vi "6517b.vi"(11 "VISA resource name":refnum<visa-resource-name>="GPIB0::12::INSTR") -> ()   [LabVIEW 2019]
uses:
  <vilib>/Utility/file.llb/Write To Spreadsheet File (DBL).vi
  lib/Keithley 6517/Keithley 6517.lvlib
panel:
  in  "Voltage Source Level (0.000000E+0)":dbl=2.0 format="%#_13g"
  in  "VISA resource name":refnum<visa-resource-name>
  in  "采集最小间隔（ms）":u32
  out "date/time string":string="20171114204549"
  in  "file path (dialog if empty)":path
  # "K"
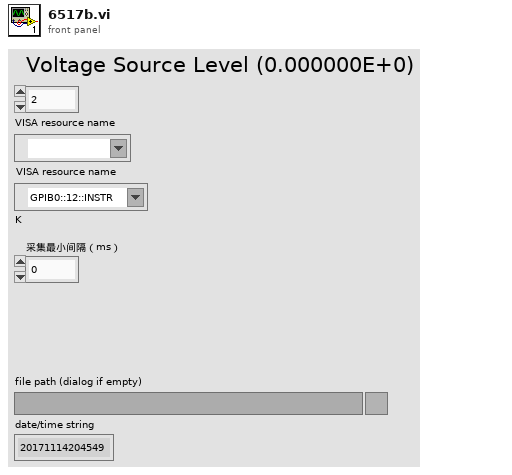
[diagram p1: front panel]
types:
  T1 = enum16{"open", "replace", "create", "open or create", "replace or create", "replace or create with confirmation"}
  T2 = cluster{"Measurement":dbl, "Units":string, "Time Stamp and Date":string, "Reading #":dbl, "Channel #":dbl}
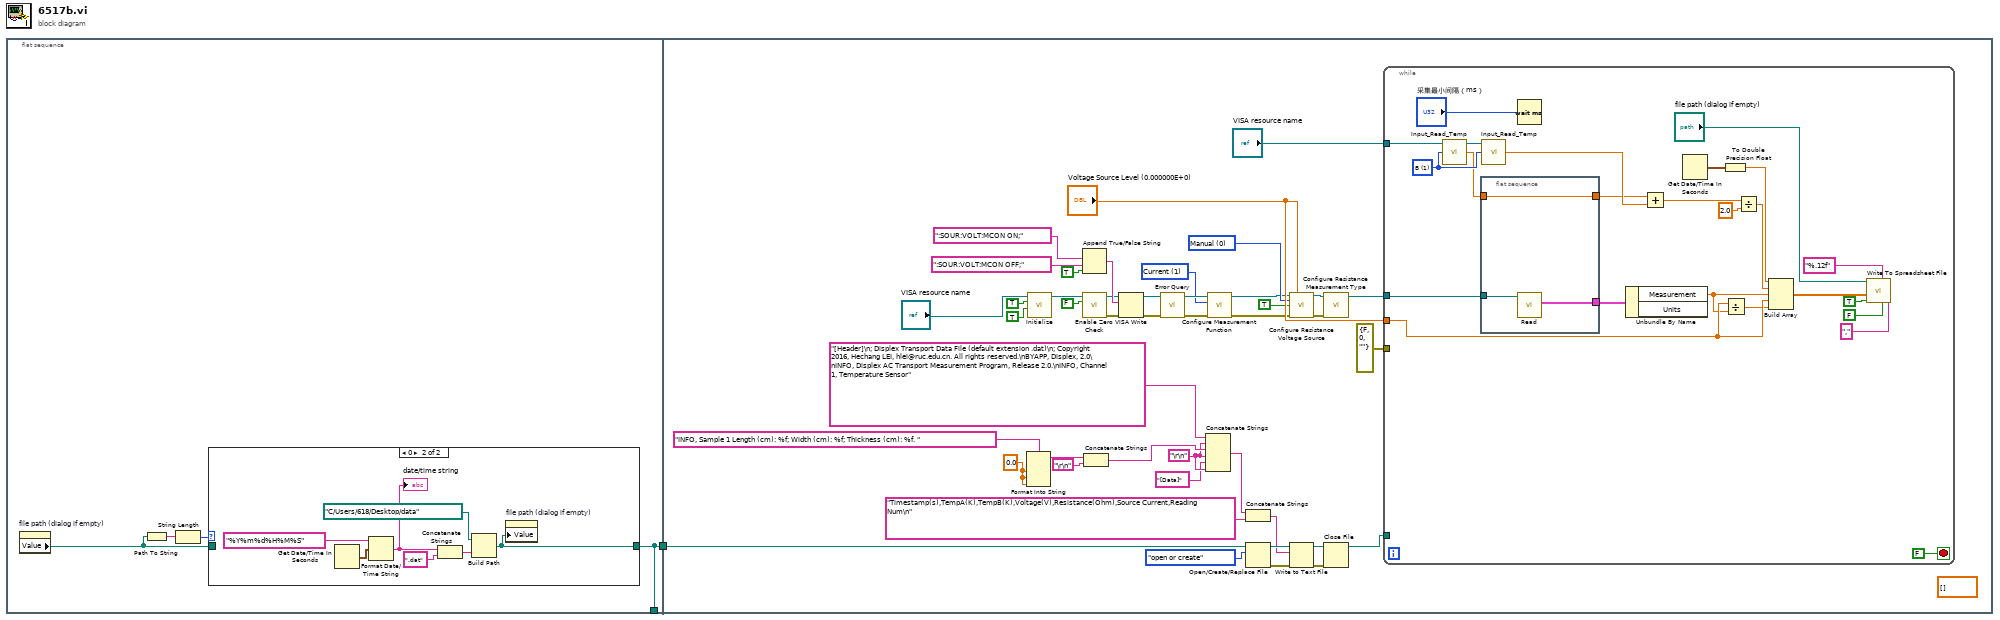
[diagram p0: block diagram]
diagram:
  n1 = flat-sequence {
    tunnel: [w2] -> _
    tunnel: [w2] -> w1
    tunnel: w1 -> [w55]
    frame #0 {
      n2 = property on="file path (dialog if empty)" class="Path"() -> ("Value"=w3:path)  [unwired: 2 in, 2 out]
      n3 = Path To String(path=w3) -> (string=w5:string)
      n4 = String Length(string=w5) -> (length=w4:i32)
      n5 = case shown="0" w4 {
        tunnel: [w6 w7] -> w2
        tunnel: w3 -> [w6 _]
        frame 1, Default {
        }
        frame 0 {
          n6 = Get Date/Time In Seconds() -> (seconds since 1Jan1904=w13:timestamp)
          n7 = Format Date/Time String(time format string (%c)="%Y%m%d%H%M%S", seconds (now)=w13) -> (date/time string=w8:string)  [unwired: 1 in]
          "date/time string" <- w8
          n8 = Concatenate Strings(w8, ".dat" ("string")) -> (w9:string)
          n9 = Build Path(base path=path "C:/Users/618/Desktop/data" ("文件夹路径"), name or relative path=w9) -> (appended path=w7:path)
          n10 = property on="file path (dialog if empty)" class="Path"("Value"=w7) -> ()  [unwired: 2 in, 2 out]
        }
      }
    }
    frame #1 {
      w18 = 1 items=["Voltage", "Current", "Resistance", "Charge"] ("Measurement Function (0: Voltage)")
      w24 = 0 items=["Manual", "Auto"] ("Voltage Source Mode (0: Manual)")
      w44 = 0.0 ("输入 1")
      w47 = "\r\n"
      (unwired) dbl[] []
      n11 = Format Into String(format string="INFO, Sample 1 Length (cm): %f; Width (cm): %f; Thickness (cm): %f. " ("string"), w44, w44, w44) -> (resulting string=w51:string)  [unwired: 2 in, 1 out]
      n12 = call "Initialize.vi"("Reset (True)"=TRUE, "ID Query (True)"=TRUE, "VISA resource name"="VISA resource name") -> ("VISA resource name out"=w16:refnum<visa-resource-name>)  [unwired: 7 in, 1 out]
      n13 = Append True/False String(1:TRUE ("Enable LO Connection (F: Disable)"), 2:":SOUR:VOLT:MCON OFF;", 3:":SOUR:VOLT:MCON ON;") -> (0:w32:string)  [unwired: 1 in]
      n14 = call "Enable Zero Check.vi"("Enable Zero Check (T: Enable)"=FALSE, "VISA resource name"=w16) -> ("error out"=w30:errorcluster, "VISA resource name out"=w31:refnum<visa-resource-name>)  [unwired: 8 in]
      n15 = Concatenate Strings(w51, "\r\n") -> (w52:string)
      n16 = VISA Write(VISA resource name=w31, write buffer=w32, error in (no error)=w30) -> (VISA resource name out=w29:refnum<visa-resource-name>, error out=w28:errorcluster)  [unwired: 1 out]
      n17 = call "Error Query.vi"("error in (no error)"=w28, "VISA resource name"=w29) -> ("error out"=w22:errorcluster, "VISA resource name out"=w21:refnum<visa-resource-name>)  [unwired: 6 in, 2 out]
      n18 = Concatenate Strings("[Header]\n; Displex Transport Data File (default extension .dat)\n; Copyright 2016, Hechang LEI, hlei@ruc.edu.cn. All rights reserved.\nBYAPP, Displex, 2.0\nINFO, Displex AC Transport Measurement Program, Release 2.0.\nINFO, Channel 1, Temperature Sensor" ("string"), w47, w52, w47, "[Data]" ("string"), w47) -> (w53:string)
      n19 = call "Configure Measurement Function.vi"("error in (no error)"=w22, "Measurement Function (0: Voltage)"=w18, "VISA resource name"=w21) -> ("error out"=w19:errorcluster, "VISA resource name out"=w20:refnum<visa-resource-name>)  [unwired: 7 in]
      n20 = Concatenate Strings(w53, "Timestamp(s),TempA(K),TempB(K),Voltage(V),Resistance(Ohm),Source Current,Reading Num\n" ("字符串")) -> (w43:string)
      n21 = Open/Create/Replace File(file path (use dialog)=w55, operation (0:open)=T1."open or create") -> (refnum out=w54:refnum<file>, error out=w40:errorcluster)  [unwired: 4 in, 1 out]
      n22 = call "Configure Resistance Voltage Source.vi"("VISA resource name"=w20, "Voltage Source Level (0.000000E+0)"="Voltage Source Level (0.000000E+0)", "Voltage Source Mode (0: Manual)"=w24, "Enable Voltage Source (F: Disable)"=TRUE, "error in (no error)"=w19) -> ("VISA resource name out"=w27:refnum<visa-resource-name>, "error out"=w26:errorcluster)  [unwired: 9 in]
      n23 = Write to Text File(file (use dialog)=w54, text=w43, error in=w40) -> (refnum out=w42:refnum<file>, error out=w41:errorcluster)  [unwired: 1 in, 1 out]
      n24 = call "Configure Resistance Measurement Type.vi"("error in (no error)"=w26, "VISA resource name"=w27) -> ("VISA resource name out"=w38:refnum<visa-resource-name>)  [unwired: 8 in, 1 out]
      n25 = Close File(refnum=w42, error in=w41) -> (path=w39:path)  [unwired: 1 out]
      n26 = while {
        tunnel: "VISA resource name" -> [w81]
        tunnel: w39 -> [_]
        tunnel: errorcluster {"status"=FALSE, "code"=0, "source"=""} ("error out") -> [_]
        tunnel: w38 -> [w70]
        tunnel: "Voltage Source Level (0.000000E+0)" -> [w61]
        stop <- FALSE stop-if-true
        w65 = u8 1 items=["A", "B", "C", "D"] ("Input")
        n27 = call "Input_Read_Temp.vi"("Input"=w65, "VISA In"=w81) -> ("Temperature"=w63:dbl, "VISA Out"=w66:refnum<visa-resource-name>)  [unwired: 1 in, 1 out]
        n28 = flat-sequence {
          tunnel: w70 -> [w84]
          tunnel: [w83] -> w64
          tunnel: w63 -> [w82]
          tunnel: [w82] -> w62
          frame #0 {
            n29 = call "Read.vi"("VISA resource name"=w84) -> ("Measurement"=w83:T2)  [unwired: 8 in, 2 out]
          }
        }
        n30 = call "Input_Read_Temp.vi"("Input"=w65, "VISA In"=w66) -> ("Temperature"=w67:dbl)  [unwired: 1 in, 2 out]
        n31 = Wait (ms)(milliseconds to wait="采集最小间隔（ms）") -> ()  [unwired: 1 out]
        n32 = Unbundle By Name(w64) -> ("Measurement"=w60:dbl)  [unwired: 1 out]
        n33 = Add(x=w62, y=w67) -> (x+y=w69:dbl)
        n34 = Get Date/Time In Seconds() -> (seconds since 1Jan1904=w75:timestamp)
        n35 = To Double Precision Float(number=w75) -> (double precision float=w74:dbl)
        n36 = Divide(x=w61, y=w60) -> (x/y=w59:dbl)
        n37 = Divide(x=w69, y=2.0) -> (x/y=w72:dbl)
        n38 = Build Array(w74, w72, w60, w61, w59) -> (w76:dbl[])
        n39 = call-poly <vilib>:"Write To Spreadsheet File.vi"("delimiter (\\t)"="," ("delimiter (\\t)"), "transpose? (no:F)"=FALSE, "format (%.3f)"="%.12f", "append to file? (new file:F)"=TRUE, "1D data"=w76, "file path (dialog if empty)"="file path (dialog if empty)") -> ()  [unwired: 2 in, 1 out]
      }
    }
  }
